vi "F Dwf Enum Device Is Opened.vi"(8 "error in (no error)":errorcluster, 10 "pfIsUsed":i32, 11 "idxDevice":i32) -> (0 "error out":errorcluster, 2 "pfIsUsed out":i32, 3 "function return":i32)   [LabVIEW 2024, in "Olasdwf.lvlib"]
doc: "DWFAPI int FDwfEnumDeviceIsOpened(int idxDevice, int *pfIsUsed);"
uses:
  Olasdwf.lvlib
  Windows/System32/dwf.dll
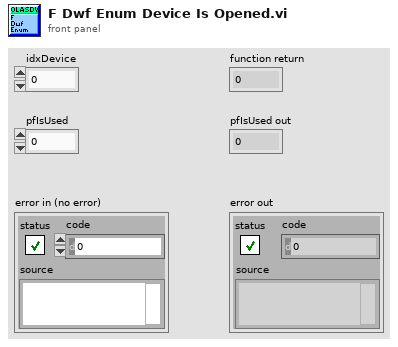
[diagram p1: front panel]
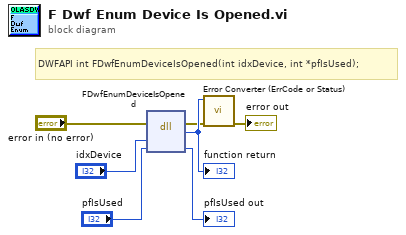
[diagram p0: block diagram]
diagram:
  # "DWFAPI int FDwfEnumDeviceIsOpened(int idxDevice, int *pfIsUsed);"
  n1 = dll-call lib="/Windows/System32/dwf.*" fn="FDwfEnumDeviceIsOpened"(error in="error in (no error)", "idxDevice"="idxDevice", "pfIsUsed"="pfIsUsed") -> (error out=w2:errorcluster, w7:i32, "pfIsUsed"=→"pfIsUsed out":i32)  [unwired: 3 in, 1 out]
  "function return" <- w7
  n2 = call "Error Converter (ErrCode or Status).vi"("error in (no error)"=w2, "error code"=w7) -> ("error out"=→"error out":errorcluster)  [unwired: 9 in]
